vi "Exponentialize Channels.vi"(2 "Channels in":dbl[](array[numeric]), 3 "Expo":dbl(slide) scale=0.0..10.0) -> (0 "Channels out":dbl[](array[numeric]))   [LabVIEW 2012]
doc: "This VI is used to apply an exponential behavior to the control input. This is similarly implemented within hobbyist scale modeling and RCs in order to replicate a more realistic or ergonomic control scheme. This improves noise reduction within the 'dead zone' of the controller interface, as such would be expected when reverting a control stick to its home position, the relative output should be significantly close to zero. By changing the 'Expo' parameter, one can adjust the severity of the exponential curve applied to the output.\nRuffin"
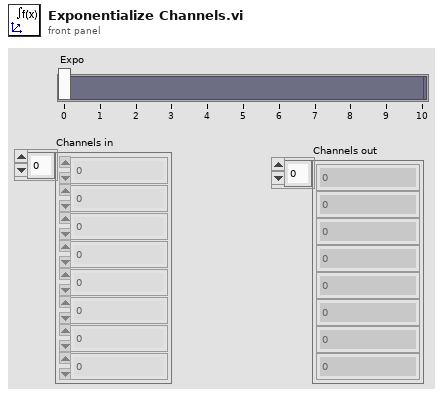
[diagram p1: front panel]
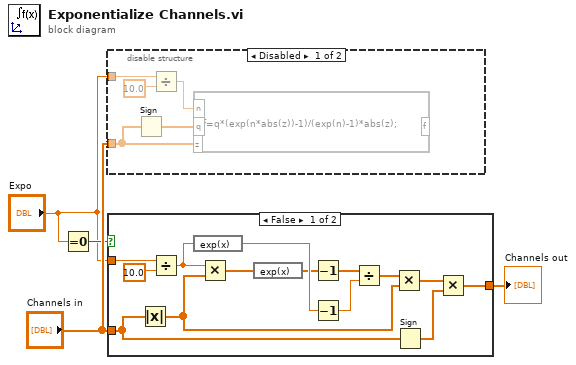
[diagram p0: block diagram]
diagram:
  n1 = Equal To 0?(x="Expo") -> (x = 0?=w2:bool)
  n2 = disable-structure shown="Disabled" {
    disable-tunnel: "Channels in" -> [w8 _]
    disable-tunnel: "Expo" -> [w7 _]
    frame Disabled {
      n3 = Sign(1:w8) -> (0:w9:dbl[])
      n4 = Divide(x=w7, y=10.0) -> (x/y=w6:dbl)
      n5 = formula code="f=q*(exp(n*abs(z))-1)/(exp(n)-1)*abs(z);"("n"=w6, "z"=w8, "q"=w9) -> ()  [unwired: 1 out]
    }
    frame Enabled {
    }
  }
  n6 = case shown="False" w2 {
    tunnel: [w17 w24] -> w4
    tunnel: "Channels in" -> [w16 w24]
    tunnel: "Expo" -> [w11 _]
    frame False {
      n7 = Absolute Value(x=w16) -> (abs(x)=w19:dbl[])
      n8 = Divide(x=w11, y=10.0) -> (x/y=w12:dbl)
      n9 = expression code="exp(x)"(w12) -> (w22:dbl)
      n10 = Multiply(x=w12, y=w19) -> (x*y=w23:dbl[])
      n11 = expression code="exp(x)"(w23) -> (w21:dbl[])
      n12 = Decrement(x=w21) -> (x-1=w20:dbl[])
      n13 = Decrement(x=w22) -> (x-1=w15:dbl)
      n14 = Divide(x=w20, y=w15) -> (x/y=w14:dbl[])
      n15 = Multiply(x=w14, y=w19) -> (x*y=w13:dbl[])
      n16 = Sign(1:w16) -> (0:w18:dbl[])
      n17 = Multiply(x=w13, y=w18) -> (x*y=w17:dbl[])
    }
    frame True {
    }
  }
  "Channels out" <- w4
